vi "GEA2 Read ERD.vi"(0 "GEA2 Reference In":refnum<k24>, 1 "Retry Count":i32=5, 2 "Read Timeout (ms)":u32=500, 5 "GEA Inputs":T2 {"Destination" format="%.0x"; "Source" format="%.0x"}, 7 "Read ERD List":T3[](array[typedef]) {"ERD Number" format="%.0x"}, 9 "GEA2 Event Registration":refnum<event-registration>, 11 "Error In":errorcluster, 13 "Verify ERD Response?":bool=TRUE) -> (4 "GEA2 Reference Out":refnum<k24>, 6 "Raw Data Out":string, 8 "ERD Data Out":T1[](array[typedef]) {"ERD Number" format="%.0x"}, 10 "Event Registration Refnum":refnum<event-registration>, 15 "Error Out":errorcluster)   [LabVIEW 2016, in "GEA2_Toolkit.lvlib"]
doc: "This VI reads an array of ERDs with a single command and returns the data in the data type selected."
uses:
  library/GEA2_Toolkit.lvlib
  type defs/ERD Read Data In.ctl
  type defs/Data Type.ctl
  type defs/Source_Destination.ctl
  type defs/ERD Read Data Out.ctl
  C:/Technology Lab/NI-2010/Trunk/Utility/LabVIEW GEA2 Toolkit v1.0.0.0/Appliance.NET/GeaCommunication.dll
  Appliance.NET/GeaCommunication.dll
  type defs/Data Out.ctl
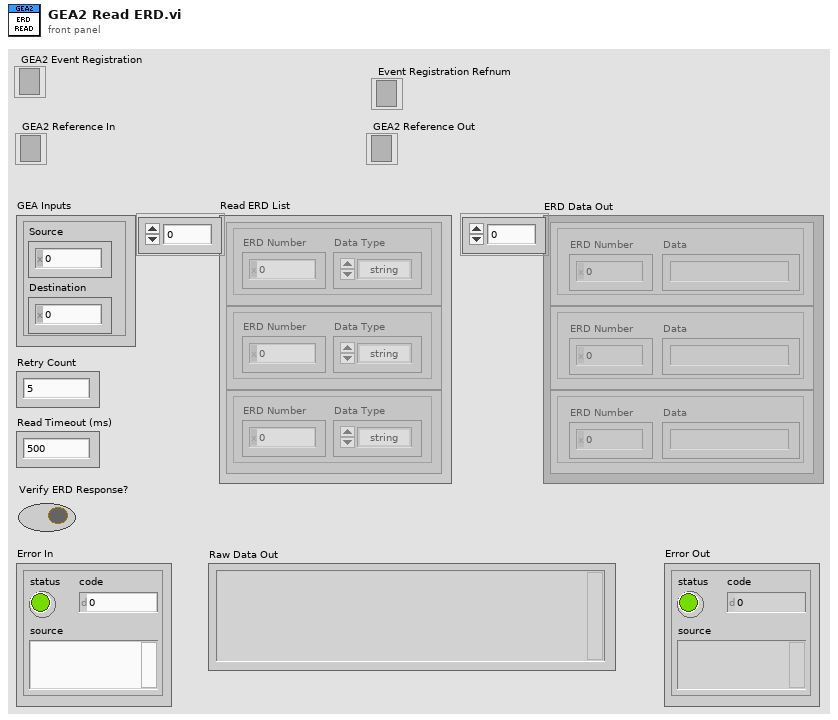
[diagram p1: front panel]
types:
  T1 = typedef "GEA2_Toolkit.lvlib/ERD Read Data Out.ctl" = cluster{"ERD Number":u16, "Data":string}
  T2 = typedef "GEA2_Toolkit.lvlib/Source_Destination.ctl" = cluster{"Source":u8, "Destination":u8}
  T3 = typedef "GEA2_Toolkit.lvlib/ERD Read Data In.ctl" = cluster{"ERD Number":u16, "Data Type":T4}
  T4 = typedef "GEA2_Toolkit.lvlib/Data Type.ctl" = enum16{"string", "boolean", "uint8_t", "uint16_t", "uint32_t", "uint64_t"}
  T5 = typedef "GEA2_Toolkit.lvlib/Data In.ctl" = cluster{"Source":u8, "Destination":u8, "Command":u8, "Message":string}
  T6 = typedef "GEA2_Toolkit.lvlib/Data Out.ctl" = cluster{"Source":u8, "Destination":u8, "Command":u8, "Length":u8, "CRC":u16, "Message":string}
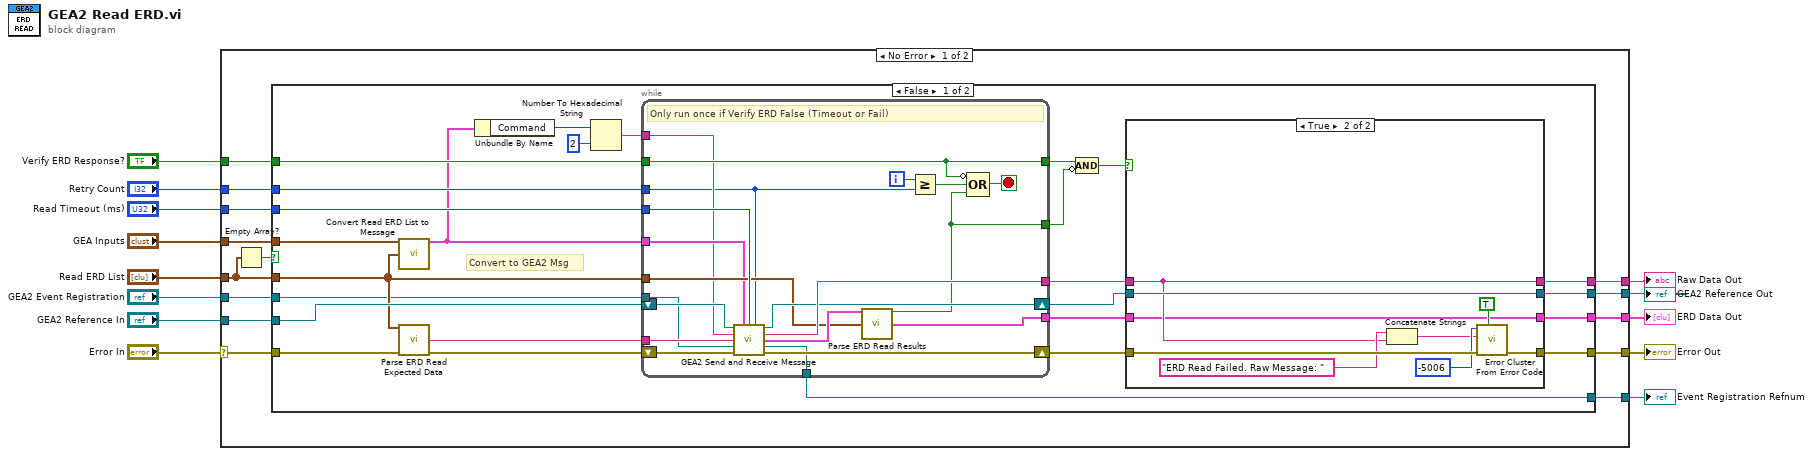
[diagram p0: block diagram]
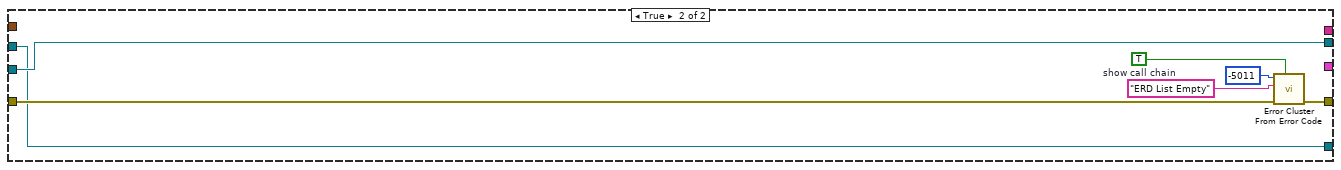
[diagram p3: hidden frame]
diagram:
  n1 = case shown="No Error" "Error In" {
    selector: "Error In" -> [w27 w95]
    tunnel: "GEA2 Reference In" -> [w26 w96]
    tunnel: "Read ERD List" -> [w17 _]
    tunnel: "Verify ERD Response?" -> [w24 _]
    tunnel: "GEA Inputs" -> [w25 _]
    tunnel: [w20 _] -> w9
    tunnel: [w21 w95] -> w8
    tunnel: "Read Timeout (ms)" -> [w23 _]
    tunnel: "Retry Count" -> [w22 _]
    tunnel: [w19 w96] -> w3
    tunnel: [w18 _] -> w5
    tunnel: "GEA2 Event Registration" -> [w15 w94]
    tunnel: [w14 w94] -> w1
    frame No Error {
      n2 = Empty Array?(array=w17) -> (empty?=w16:bool)
      n3 = case shown="False" w16 {
        tunnel: w27 -> [w36 w90]
        tunnel: w26 -> [w53 w88]
        tunnel: w25 -> [w52 _]
        tunnel: w24 -> [w51 _]
        tunnel: w23 -> [w50 _]
        tunnel: w22 -> [w49 _]
        tunnel: [w47 w89] -> w21
        tunnel: [w46 _] -> w20
        tunnel: [w43 w88] -> w19
        tunnel: [w42 _] -> w18
        tunnel: w17 -> [w37 _]
        tunnel: w15 -> [w29 w87]
        tunnel: [w28 w87] -> w14
        frame False {
          # "Convert to GEA2 Msg"
          n4 = call "Convert Read ERD List to Message.vi"("GEA Inputs"=w52, "Read ERD List"=w37) -> ("GEA Message"=w32:T5)  [unwired: 12 in, 1 out]
          n5 = call "Parse ERD Read Expected Data.vi"("Read ERD List"=w37, "Error In"=w36) -> ("Expected Data"=w35:string, "Error Out"=w34:errorcluster)  [unwired: 12 in]
          n6 = Unbundle By Name(w32) -> ("Command"=w31:u8)
          n7 = Number To Hexadecimal String(1:i16 2 ("width (-)"), 2:w31) -> (0:w30:string)
          n8 = while {
            tunnel: w32 -> [w71]
            tunnel: [w86] -> w45
            tunnel: w51 -> [w80]
            tunnel: w37 -> [w76]
            tunnel: [w78] -> w41
            tunnel: w50 -> [w84]
            tunnel: w49 -> [w67]
            tunnel: [w80] -> w39
            tunnel: [w74] -> w38
            tunnel: w35 -> [w73]
            shift-right: [w85] -> w48
            shift-left: w34 -> [w72]
            shift-right: [w81] -> w44
            shift-left: w53 -> [w79]
            tunnel: w30 -> [w70]
            tunnel: w29 -> [w69]
            tunnel: [w68] -> w28
            i -> [w83]
            stop <- w82 stop-if-true
            # "Only run once if Verify ERD False (Timeout or Fail)"
            n9 = call "GEA2 Send and Receive Message.vi"("GEA2 Reference In"=w79, "Input Data"=w71, "Read Timeout (ms)"=w84, "# of Retries"=w67, "Expected Command"=w70, "Expected Data"=w73, "GEA2 Event Registration"=w69, "Error In"=w72) -> ("GEA2 Reference Out"=w81:refnum<k24>, "Raw Data Out"=w86:string, "Converted Data Out"=w77:T6, "Event Registration Out"=w68:refnum<event-registration>, "Error Out"=w85:errorcluster)  [unwired: 2 in, 1 out]
            n10 = call "Parse ERD Read Results.vi"("Converted Data"=w77, "Read ERD List"=w76) -> ("Pass/Fail?"=w74:bool, "ERD Data Out"=w78:T1[])  [unwired: 12 in]
            n11 = Greater Or Equal?(x=w83, y=w67) -> (x >= y?=w75:bool)
            n12 = Compound Arithmetic op=OR(invert w80, w75, w74) -> (w82:bool)
          }
          n13 = Compound Arithmetic op=AND(w39, invert w38) -> (w40:bool)
          n14 = case shown="True" w40 {
            tunnel: w48 -> [w57 w66]
            tunnel: [w57 w65] -> w47
            tunnel: [w56 w59] -> w46
            tunnel: w45 -> [w56 w59]
            tunnel: w44 -> [w55 w62]
            tunnel: [w55 w62] -> w43
            tunnel: [w54 w58] -> w42
            tunnel: w41 -> [w54 w58]
            frame False {
              # "If Verify ERD True & (Timeout or Fail occurred) -> Create Error"
            }
            frame True {
              n15 = Concatenate Strings("ERD Read Failed. Raw Message: " ("error message (\"\")"), w59) -> (w60:string)
              n16 = call <vilib>:"Error Cluster From Error Code.vi"("show call chain? (False)"=TRUE, "error in (no error)"=w66, "error message (\"\")"=w60, "error code (0)"=-5006) -> ("error out"=w65:errorcluster)  [unwired: 5 in]
            }
          }
        }
        frame True {
          w91 = TRUE  # show call chain
          n17 = call <vilib>:"Error Cluster From Error Code.vi"("show call chain? (False)"=w91, "error in (no error)"=w90, "error message (\"\")"="ERD List Empty" ("error message (\"\")"), "error code (0)"=-5011) -> ("error out"=w89:errorcluster)  [unwired: 5 in]
        }
      }
    }
    frame Error {
    }
  }
  "Raw Data Out" <- w9
  "Error Out" <- w8
  "ERD Data Out" <- w5
  "GEA2 Reference Out" <- w3
  "Event Registration Refnum" <- w1
